vi "CSM_GNSS.vi"(8 "Error In":errorcluster, 11 "Command":string) -> (0 "Error Out":errorcluster, 3 "Response":string)   [LabVIEW 2018]
uses:
  MOKO_LabViewLibrary/MokoLowLevel/MokoLowLovelControl/MLLC_Mode.ctl
  data/CSM_GNSS.ctl
  windows/Environments.ctl
  windows/Equipment.ctl
  windows/Registration.ctl
panel:
  in  "Settings":T5
  in  "Error Code":u32
  in  "Utility Name":string="CSM_GNSS"
  in  "Mode":T6
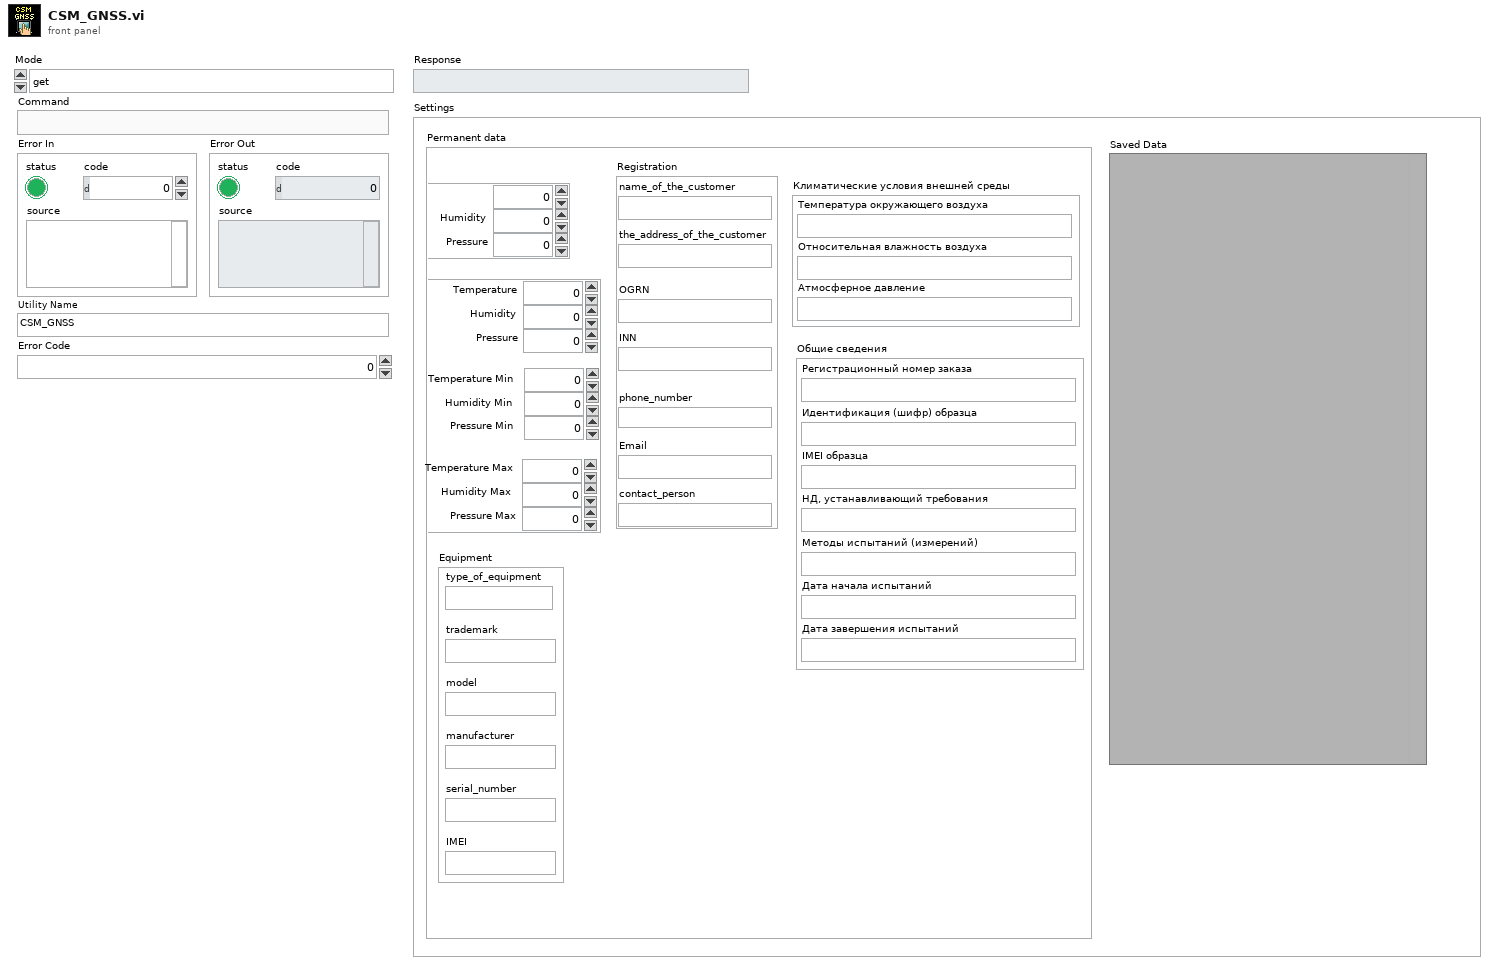
[diagram p1: front panel]
types:
  T1 = typedef "CSM_GNSS.ctl" = cluster{"Environment":cluster{"Temperature":dbl, "Humidity":dbl, "Pressure":dbl}, "Environments":T2, "Equipment":T3, "Registration":T4, "Общие сведения":cluster{"Регистрационный номер заказа":string, "Идентификация (шифр) образца":string, "IMEI образца":string, "НД, устанавливающий требования":string, "Методы испытаний (измерений)":string, "Дата начала испытаний":string, "Дата завершения испытаний":string}, "Климатические условия внешней среды":cluster{"Температура окружающего воздуха":string, "Относительная влажность воздуха":string, "Атмосферное давление":string}}
  T2 = typedef "Environments.ctl" = cluster{"Temperature Min":dbl, "Humidity Min":dbl, "Pressure Min":dbl, "Temperature Max":dbl, "Humidity Max":dbl, "Pressure Max":dbl, "Temperature":dbl, "Humidity":dbl, "Pressure":dbl}
  T3 = typedef "Equipment.ctl" = cluster{"type_of_equipment":string, "trademark":string, "model":string, "manufacturer":string, "serial_number":string, "IMEI":string}
  T4 = typedef "Registration.ctl" = cluster{"name_of_the_customer":string, "the_address_of_the_customer":string, "OGRN":string, "INN":string, "phone_number":string, "Email":string, "contact_person":string}
  T5 = cluster{"Permanent data":T1, "Saved Data":variant}
  T6 = typedef "MLLC_Mode.ctl" = enum16{"get", "set", "close", "Init", "Check"}
  T7 = cluster{"Temperature":dbl, "Humidity":dbl, "Pressure":dbl}
  T8 = typedef "MLLC_Error.ctl" = errorcluster
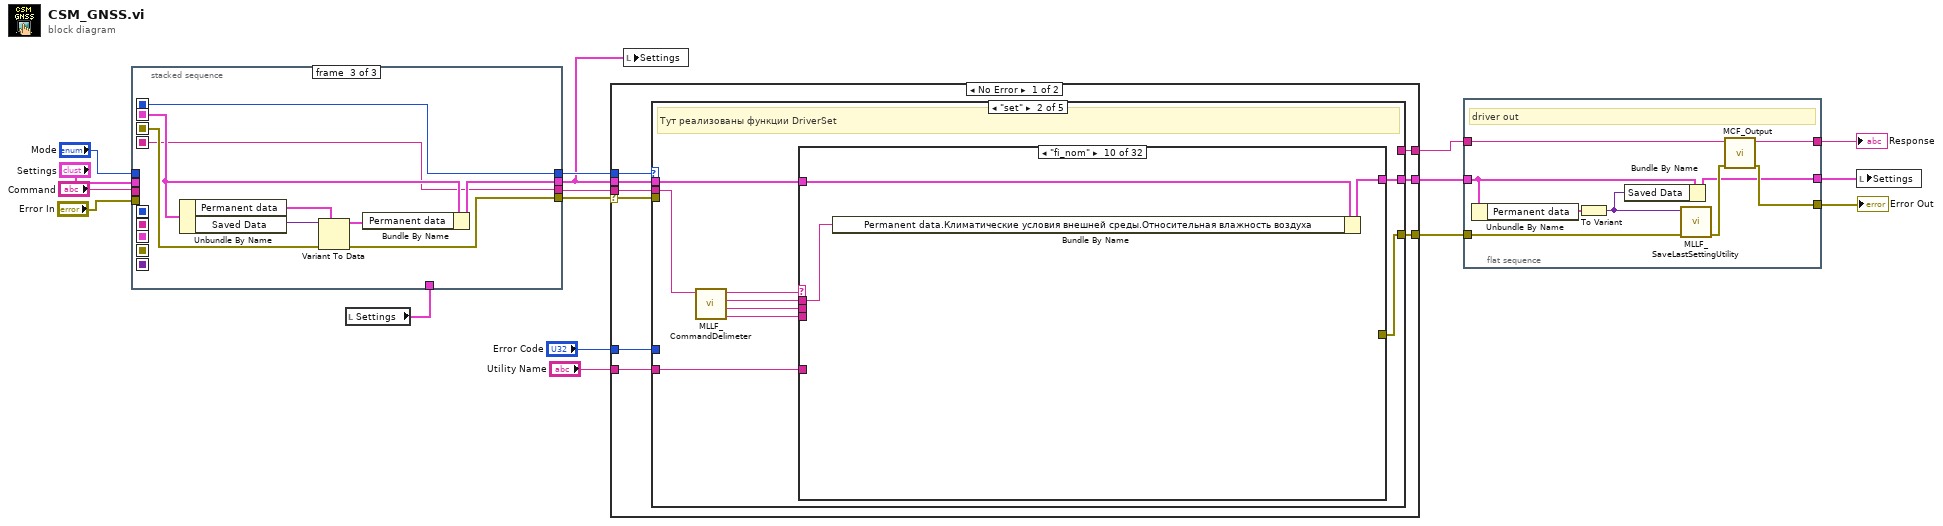
[diagram p0: block diagram]
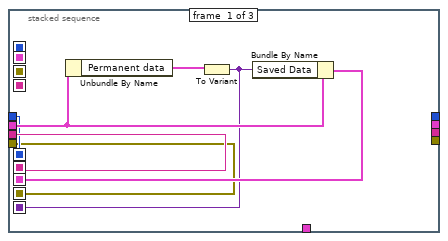
[diagram p2: hidden frame]
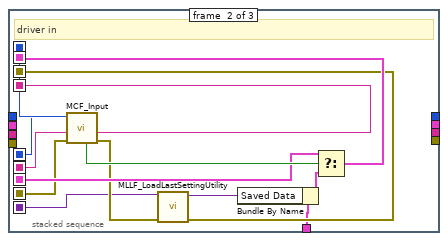
[diagram p3: hidden frame]
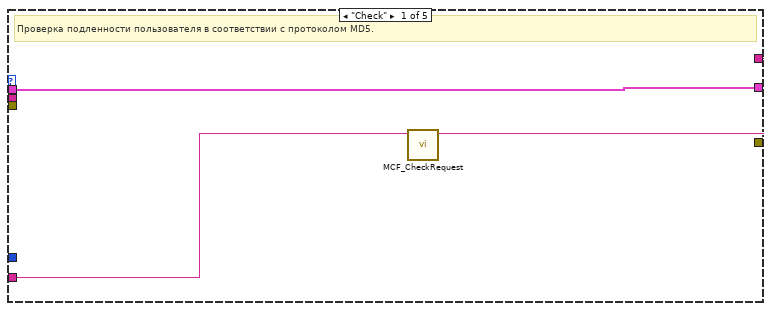
[diagram p4: hidden frame]
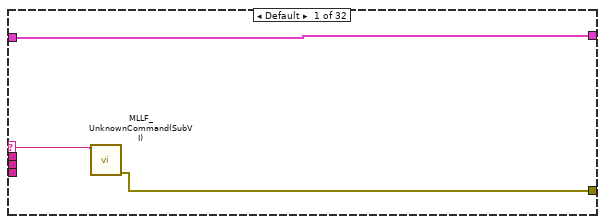
[diagram p5: hidden frame]
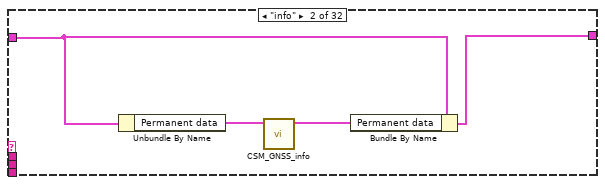
[diagram p6: hidden frame]
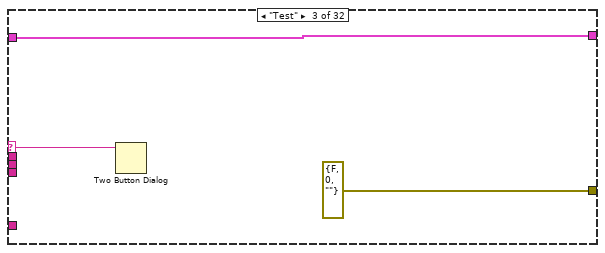
[diagram p7: hidden frame]
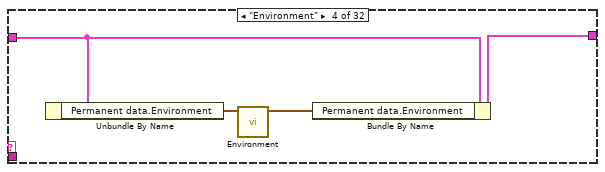
[diagram p8: hidden frame]
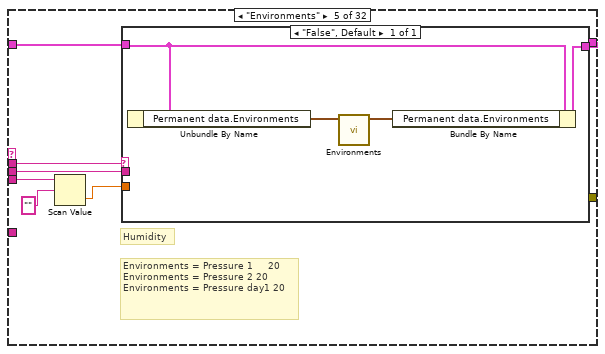
[diagram p9: hidden frame]
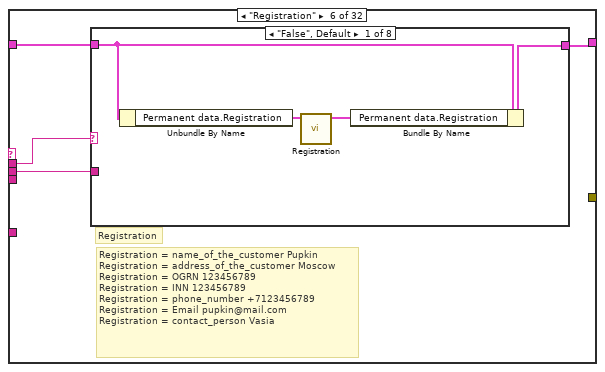
[diagram p10: hidden frame]
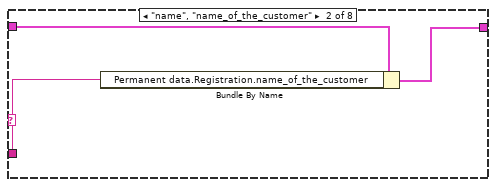
[diagram p11: hidden frame]
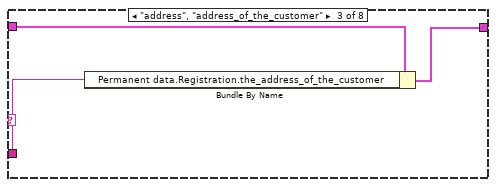
[diagram p12: hidden frame]
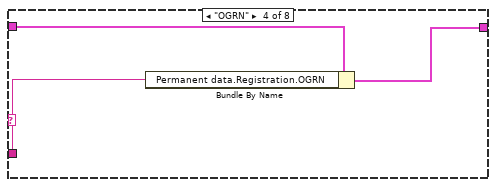
[diagram p13: hidden frame]
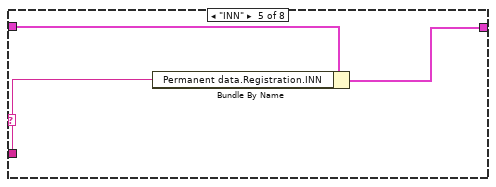
[diagram p14: hidden frame]
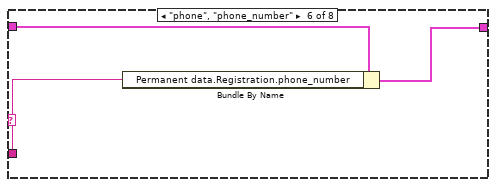
[diagram p15: hidden frame]
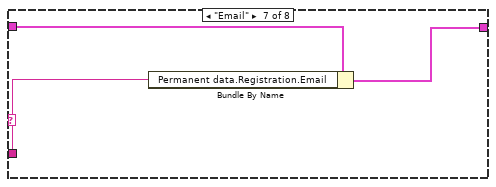
[diagram p16: hidden frame]
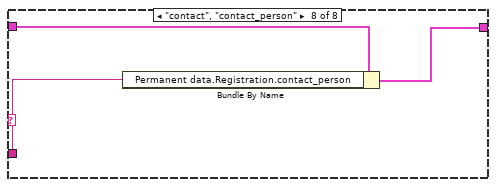
[diagram p17: hidden frame]
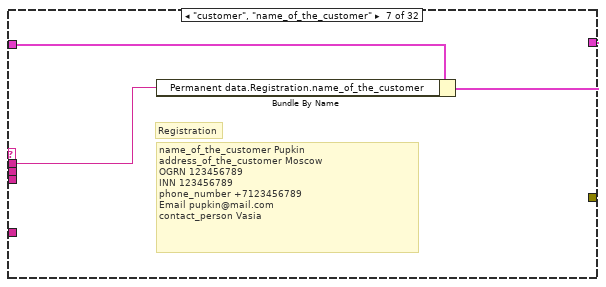
[diagram p18: hidden frame]
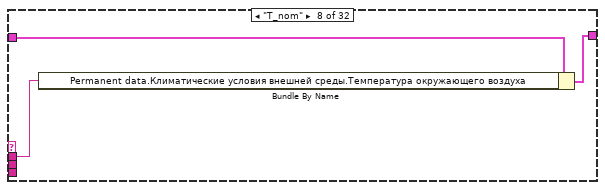
[diagram p19: hidden frame]
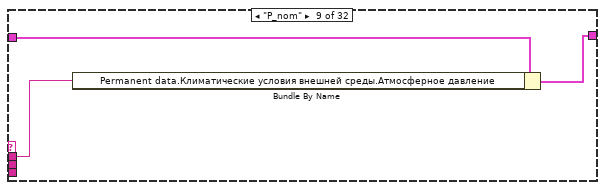
[diagram p20: hidden frame]
diagram:
  n1 = local read "Settings"() -> (w11:T5)
  n2 = stacked-sequence {
    seq-local: [w20 _ _] -> [_ w36 _]
    seq-local: [w19 _ _] -> [_ w37 _]
    seq-local: [w22 _ _] -> [_ w32 _]
    seq-local: [w18 _ _] -> [_ w31 _]
    seq-local: [w21 _ _] -> [_ w26 _]
    seq-local: [_ w27 _] -> [_ _ w43]
    seq-local: [_ w38 _] -> [_ _ w40]
    seq-local: [_ w35 _] -> [_ _ w39]
    seq-local: [_ w34 _] -> [_ _ w44]
    tunnel: "Command" -> [w20 _ _]
    tunnel: "Mode" -> [w19 _ _]
    tunnel: "Error In" -> [w18 _ _]
    tunnel: "Settings" -> [w23 _ _]
    tunnel: w11 -> [_ w25 _]
    tunnel: [_ _ w39] -> w7
    tunnel: [_ _ w42] -> w9
    tunnel: [_ _ w41] -> w8
    tunnel: [_ _ w40] -> w10
    frame #0 {
      n3 = Unbundle By Name(w23) -> ("Permanent data"=w24:T1)
      n4 = To Variant(anything=w24) -> (Variant=w21:variant)
      n5 = Bundle By Name(cluster=w23, "Saved Data"=w21) -> (w22:T5)
    }
    frame #1 {
      # "driver in"
      n6 = call "MCF_Input.vi"("Error In"=w31, "Command in"=w36, "Mode in"=w37) -> ("Error Out"=w30:errorcluster, "Command out"=w35:string, "Mode out"=w38:T6, "Boolean"=w33:bool)  [unwired: 5 in]
      n7 = call "MLLF_LoadLastSettingUtility.vi"("Error In"=w30, "Save data in"=w26) -> ("Error Out"=w27:errorcluster, "Save data out"=w29:variant)  [unwired: 8 in]
      n8 = Bundle By Name(cluster=w25, "Saved Data"=w29) -> (w28:T5)
      n9 = Select(t=w32, s=w33, f=w28) -> (s? t:f=w34:T5)
    }
    frame #2 {
      n10 = Unbundle By Name(w44) -> ("Permanent data"=w45:T1, "Saved Data"=w47:variant)
      n11 = Variant To Data(error in=w43, type=w45, Variant=w47) -> (data=w46:T1, error out=w41:errorcluster)
      n12 = Bundle By Name(cluster=w44, "Permanent data"=w46) -> (w42:T5)
    }
  }
  n13 = case shown="No Error" w8 {
    selector: w8 -> [w52 w346]
    tunnel: [w54 w346] -> w4
    tunnel: w10 -> [w56 _]
    tunnel: [w55 _] -> w6
    tunnel: w7 -> [w53 _]
    tunnel: w9 -> [w49 w345]
    tunnel: "Error Code" -> [w51 _]
    tunnel: "Utility Name" -> [w50 _]
    tunnel: [w48 w345] -> w5
    frame No Error {
      n14 = case shown="\"set\"" w56 {
        tunnel: [w57 _ w221 _ _] -> w55
        tunnel: [_ w67 w223 _ _] -> w54
        tunnel: w53 -> [_ w68 w226 _ _]
        tunnel: w52 -> [_ _ _ _ _]
        tunnel: w51 -> [_ _ _ _ _]
        tunnel: w50 -> [w58 w60 w220 _ _]
        tunnel: w49 -> [w59 w66 w225 _ _]
        tunnel: [w59 w65 w224 _ _] -> w48
        frame "Check" {
          # "Проверка подленности пользователя в соответствии с протоколом MD5."
          n15 = call "MCF_CheckRequest.vi"("Driver Name"=w58) -> ("Output String"=w57:string)  [unwired: 9 in, 1 out]
        }
        frame "set" {
          # "Тут реализованы функции DriverSet"
          n16 = call "MLLF_CommandDelimeter.vi"("command with param"=w68) -> ("param 3"=w61:string, "param 2"=w62:string, "param 1"=w64:string, "command"=w63:string)  [unwired: 6 in, 1 out]
          n17 = case shown="\"fi_nom\"" w63 {
            selector: w63 -> [w70 _ w76 _ _ _ _ _ _ _ _ _ _ _ _ _ _ _ _ _ _ _ _ _ _ _ _ _ _ _ _ _]
            tunnel: [w71 w72 w78 w80 w88 w96 w124 w127 w130 w133 w136 w139 w142 w145 w148 w151 w153 w158 w161 w164 w167 w170 w173 w178 w183 w188 w193 w198 w203 w208 w213 w218] -> w65
            tunnel: w66 -> [w71 w74 w78 w81 w89 w97 w125 w128 w131 w134 w137 w140 w143 w146 w149 w152 w155 w159 w162 w165 w168 w171 w174 w179 w184 w189 w194 w199 w204 w209 w214 w219]
            tunnel: [w69 _ errorcluster {"status"=FALSE, "code"=0, "source"=""} ("error IO") _ _ _ _ _ _ _ _ _ _ _ _ _ _ _ _ _ _ _ _ _ _ _ _ _ _ _ _ _] -> w67
            tunnel: w64 -> [_ _ _ _ w85 w95 w123 w126 w129 w132 w135 w138 w141 w144 w147 w150 _ w157 w160 w163 w166 w169 w172 w175 w180 w185 w190 w195 w200 w205 w210 w215]
            tunnel: w62 -> [_ _ _ _ w84 w94 _ _ _ _ _ _ _ _ _ _ _ _ _ _ _ _ _ _ _ _ _ _ _ _ _ _]
            tunnel: w61 -> [_ _ _ _ w83 _ _ _ _ _ _ _ _ _ _ _ _ _ _ _ _ _ _ _ _ _ _ _ _ _ _ _]
            tunnel: w60 -> [_ _ _ _ _ _ _ _ _ _ _ _ _ _ _ _ _ _ _ _ _ _ _ _ _ _ _ _ _ _ _ _]
            frame Default {
              n18 = call "MLLF_UnknownCommand(SubVI).vi"("Unknown command"=w70) -> ("error out"=w69:errorcluster)  [unwired: 10 in]
            }
            frame "info" {
              n19 = Unbundle By Name(w74) -> ("Permanent data"=w75:T1)
              n20 = call "CSM_GNSS_info.vi"("CSMinfo in"=w75) -> ("CSMinfo out"=w73:T1)  [unwired: 9 in, 1 out]
              n21 = Bundle By Name(cluster=w74, "Permanent data"=w73) -> (w72:T5)
            }
            frame "Test" {
              n22 = Two Button Dialog(message=w76) -> ()  [unwired: 2 in, 1 out]
            }
            frame "Environment" {
              n23 = Unbundle By Name(w81) -> ("Permanent data.Environment"=w82:T7)
              n24 = call "Environment.vi"("Environment in"=w82) -> ("Environment out"=w79:T7)  [unwired: 9 in, 1 out]
              n25 = Bundle By Name(cluster=w81, "Permanent data.Environment"=w79) -> (w80:T5)
            }
            frame "Environments" {
              # "Humidity"
              # "Environments = Pressure 1     20\nEnvironments = Pressure 2 20\nEnvironments = Pressure day1 20"
              n26 = Scan Value(string=w83, format string="") -> (value=w87:dbl)  [unwired: 1 in, 1 out]
              n27 = case shown="\"False\", Default" w85 {
                tunnel: w89 -> [w91]
                tunnel: [w90] -> w88
                tunnel: w87 -> [_]
                tunnel: w84 -> [_]
                frame "False", Default {
                  n28 = Unbundle By Name(w91) -> ("Permanent data.Environments"=w93:T2)
                  n29 = call "Environments.vi"("Environments in"=w93) -> ("Environments out"=w92:T2)  [unwired: 9 in, 1 out]
                  n30 = Bundle By Name(cluster=w91, "Permanent data.Environments"=w92) -> (w90:T5)
                }
              }
            }
            frame "Registration" {
              # "Registration"
              # "Registration = name_of_the_customer Pupkin\nRegistration = address_of_the_customer Moscow\nRegistration = OGRN 123456789\nRegistration = INN 123456789\nRegistration = phone_number +7123456789\nRegistration = Email pupkin@mail.com\nRegistration = contact_person Vasia"
              n31 = case shown="\"False\", Default" w95 {
                tunnel: w97 -> [w100 w104 w107 w110 w113 w116 w119 w122]
                tunnel: [w99 w103 w106 w109 w112 w115 w118 w121] -> w96
                tunnel: w94 -> [_ w102 w105 w108 w111 w114 w117 w120]
                frame "False", Default {
                  n32 = Unbundle By Name(w100) -> ("Permanent data.Registration"=w101:T4)
                  n33 = call "Registration.vi"("Registration in"=w101) -> ("Registration out"=w98:T4)  [unwired: 9 in, 1 out]
                  n34 = Bundle By Name(cluster=w100, "Permanent data.Registration"=w98) -> (w99:T5)
                }
                frame "name", "name_of_the_customer" {
                  n35 = Bundle By Name(cluster=w104, "Permanent data.Registration.name_of_the_customer"=w102) -> (w103:T5)
                }
                frame "address", "address_of_the_customer" {
                  n36 = Bundle By Name(cluster=w107, "Permanent data.Registration.the_address_of_the_customer"=w105) -> (w106:T5)
                }
                frame "OGRN" {
                  n37 = Bundle By Name(cluster=w110, "Permanent data.Registration.OGRN"=w108) -> (w109:T5)
                }
                frame "INN" {
                  n38 = Bundle By Name(cluster=w113, "Permanent data.Registration.INN"=w111) -> (w112:T5)
                }
                frame "phone", "phone_number" {
                  n39 = Bundle By Name(cluster=w116, "Permanent data.Registration.phone_number"=w114) -> (w115:T5)
                }
                frame "Email" {
                  n40 = Bundle By Name(cluster=w119, "Permanent data.Registration.Email"=w117) -> (w118:T5)
                }
                frame "contact", "contact_person" {
                  n41 = Bundle By Name(cluster=w122, "Permanent data.Registration.contact_person"=w120) -> (w121:T5)
                }
              }
            }
            frame "customer", "name_of_the_customer" {
              # "Registration"
              # "name_of_the_customer Pupkin\naddress_of_the_customer Moscow\nOGRN 123456789\nINN 123456789\nphone_number +7123456789\nEmail pupkin@mail.com\ncontact_person Vasia"
              n42 = Bundle By Name(cluster=w125, "Permanent data.Registration.name_of_the_customer"=w123) -> (w124:T5)
            }
            frame "T_nom" {
              n43 = Bundle By Name(cluster=w128, "Permanent data.Климатические условия внешней среды.Температура окружающего воздуха"=w126) -> (w127:T5)
            }
            frame "P_nom" {
              n44 = Bundle By Name(cluster=w131, "Permanent data.Климатические условия внешней среды.Атмосферное давление"=w129) -> (w130:T5)
            }
            frame "fi_nom" {
              n45 = Bundle By Name(cluster=w134, "Permanent data.Климатические условия внешней среды.Относительная влажность воздуха"=w132) -> (w133:T5)
            }
            frame "address", "the_address_of_the_customer" {
              # "Registration"
              # "name_of_the_customer Pupkin\naddress_of_the_customer Moscow\nOGRN 123456789\nINN 123456789\nphone_number +7123456789\nEmail pupkin@mail.com\ncontact_person Vasia"
              n46 = Bundle By Name(cluster=w137, "Permanent data.Registration.the_address_of_the_customer"=w135) -> (w136:T5)
            }
            frame "OGRN" {
              # "Registration"
              # "name_of_the_customer Pupkin\naddress_of_the_customer Moscow\nOGRN 123456789\nINN 123456789\nphone_number +7123456789\nEmail pupkin@mail.com\ncontact_person Vasia"
              n47 = Bundle By Name(cluster=w140, "Permanent data.Registration.OGRN"=w138) -> (w139:T5)
            }
            frame "INN" {
              # "Registration"
              # "name_of_the_customer Pupkin\naddress_of_the_customer Moscow\nOGRN 123456789\nINN 123456789\nphone_number +7123456789\nEmail pupkin@mail.com\ncontact_person Vasia"
              n48 = Bundle By Name(cluster=w143, "Permanent data.Registration.INN"=w141) -> (w142:T5)
            }
            frame "phone", "phone_number" {
              # "Registration"
              # "name_of_the_customer Pupkin\naddress_of_the_customer Moscow\nOGRN 123456789\nINN 123456789\nphone_number +7123456789\nEmail pupkin@mail.com\ncontact_person Vasia"
              n49 = Bundle By Name(cluster=w146, "Permanent data.Registration.phone_number"=w144) -> (w145:T5)
            }
            frame "Email" {
              # "Registration"
              # "name_of_the_customer Pupkin\naddress_of_the_customer Moscow\nOGRN 123456789\nINN 123456789\nphone_number +7123456789\nEmail pupkin@mail.com\ncontact_person Vasia"
              n50 = Bundle By Name(cluster=w149, "Permanent data.Registration.Email"=w147) -> (w148:T5)
            }
            frame "contact", "contact_person" {
              # "Registration"
              # "name_of_the_customer Pupkin\naddress_of_the_customer Moscow\nOGRN 123456789\nINN 123456789\nphone_number +7123456789\nEmail pupkin@mail.com\ncontact_person Vasia"
              n51 = Bundle By Name(cluster=w152, "Permanent data.Registration.contact_person"=w150) -> (w151:T5)
            }
            frame "Equipment" {
              n52 = Unbundle By Name(w155) -> ("Permanent data.Equipment"=w156:T3)
              n53 = call "Equipment.vi"("Equipment in"=w156) -> ("Equipment out"=w154:T3)  [unwired: 9 in, 1 out]
              n54 = Bundle By Name(cluster=w155, "Permanent data.Equipment"=w154) -> (w153:T5)
            }
            frame "type_of_equipment" {
              # "Equipment"
              # "type_of_equipment Reciever\ntrademark Roga&Kopyta\nmodel Model_1\nmanufacturer Roga&Kopyta\nserial_number 123456789\nIMEI 55613216568486483465"
              n55 = Bundle By Name(cluster=w159, "Permanent data.Equipment.type_of_equipment"=w157) -> (w158:T5)
            }
            frame "trademark" {
              # "Equipment"
              # "type_of_equipment Reciever\ntrademark Roga&Kopyta\nmodel Model_1\nmanufacturer Roga&Kopyta\nserial_number 123456789\nIMEI 55613216568486483465"
              n56 = Bundle By Name(cluster=w162, "Permanent data.Equipment.trademark"=w160) -> (w161:T5)
            }
            frame "model" {
              # "Equipment"
              # "type_of_equipment Reciever\ntrademark Roga&Kopyta\nmodel Model_1\nmanufacturer Roga&Kopyta\nserial_number 123456789\nIMEI 55613216568486483465"
              n57 = Bundle By Name(cluster=w165, "Permanent data.Equipment.model"=w163) -> (w164:T5)
            }
            frame "manufacturer" {
              # "Equipment"
              # "type_of_equipment Reciever\ntrademark Roga&Kopyta\nmodel Model_1\nmanufacturer Roga&Kopyta\nserial_number 123456789\nIMEI 55613216568486483465"
              n58 = Bundle By Name(cluster=w168, "Permanent data.Equipment.manufacturer"=w166) -> (w167:T5)
            }
            frame "serial_number" {
              # "Equipment"
              # "type_of_equipment Reciever\ntrademark Roga&Kopyta\nmodel Model_1\nmanufacturer Roga&Kopyta\nserial_number 123456789\nIMEI 55613216568486483465"
              n59 = Bundle By Name(cluster=w171, "Permanent data.Equipment.serial_number"=w169) -> (w170:T5)
            }
            frame "IMEI" {
              # "Equipment"
              # "type_of_equipment Reciever\ntrademark Roga&Kopyta\nmodel Model_1\nmanufacturer Roga&Kopyta\nserial_number 123456789\nIMEI 55613216568486483465"
              n60 = Bundle By Name(cluster=w174, "Permanent data.Equipment.IMEI"=w172) -> (w173:T5)
            }
            frame "Temperature" {
              # "Enviroments"
              # "Temperature 25\nHumidity 50\nPressure 100\nTemperature_min 25\nHumidity_min 50\nPressure_min 100\nTemperature_max 25\nHumidity_max 50\nPressure_max 100"
              n61 = Scan Value(string=w175, format string="") -> (value=w177:dbl)  [unwired: 1 in, 1 out]
              n62 = Bundle By Name(cluster=w179, "Permanent data.Environment.Temperature"=w177) -> (w178:T5)
            }
            frame "Humidity" {
              # "Enviroments"
              # "Temperature 25\nHumidity 50\nPressure 100\nTemperature_min 25\nHumidity_min 50\nPressure_min 100\nTemperature_max 25\nHumidity_max 50\nPressure_max 100"
              n63 = Scan Value(string=w180, format string="") -> (value=w182:dbl)  [unwired: 1 in, 1 out]
              n64 = Bundle By Name(cluster=w184, "Permanent data.Environment.Humidity"=w182) -> (w183:T5)
            }
            frame "Pressure" {
              # "Enviroments"
              # "Temperature 25\nHumidity 50\nPressure 100\nTemperature_min 25\nHumidity_min 50\nPressure_min 100\nTemperature_max 25\nHumidity_max 50\nPressure_max 100"
              n65 = Scan Value(string=w185, format string="") -> (value=w187:dbl)  [unwired: 1 in, 1 out]
              n66 = Bundle By Name(cluster=w189, "Permanent data.Environment.Pressure"=w187) -> (w188:T5)
            }
            frame "Temperature_min", "TemperatureMin" {
              # "Enviroments"
              # "Temperature 25\nHumidity 50\nPressure 100\nTemperature_min 25\nHumidity_min 50\nPressure_min 100\nTemperature_max 25\nHumidity_max 50\nPressure_max 100"
              n67 = Scan Value(string=w190, format string="") -> (value=w192:dbl)  [unwired: 1 in, 1 out]
              n68 = Bundle By Name(cluster=w194, "Permanent data.Environments.Temperature Min"=w192) -> (w193:T5)
            }
            frame "Humidity_min", "HumidityMin" {
              # "Enviroments"
              # "Temperature 25\nHumidity 50\nPressure 100\nTemperature_min 25\nHumidity_min 50\nPressure_min 100\nTemperature_max 25\nHumidity_max 50\nPressure_max 100"
              n69 = Scan Value(string=w195, format string="") -> (value=w197:dbl)  [unwired: 1 in, 1 out]
              n70 = Bundle By Name(cluster=w199, "Permanent data.Environments.Humidity Min"=w197) -> (w198:T5)
            }
            frame "Pressure_min", "PressureMin" {
              # "Enviroments"
              # "Temperature 25\nHumidity 50\nPressure 100\nTemperature_min 25\nHumidity_min 50\nPressure_min 100\nTemperature_max 25\nHumidity_max 50\nPressure_max 100"
              n71 = Scan Value(string=w200, format string="") -> (value=w202:dbl)  [unwired: 1 in, 1 out]
              n72 = Bundle By Name(cluster=w204, "Permanent data.Environments.Pressure Min"=w202) -> (w203:T5)
            }
            frame "Temperature_max", "TemperatureMax" {
              # "Enviroments"
              # "Temperature 25\nHumidity 50\nPressure 100\nTemperature_min 25\nHumidity_min 50\nPressure_min 100\nTemperature_max 25\nHumidity_max 50\nPressure_max 100"
              n73 = Scan Value(string=w205, format string="") -> (value=w207:dbl)  [unwired: 1 in, 1 out]
              n74 = Bundle By Name(cluster=w209, "Permanent data.Environments.Temperature Max"=w207) -> (w208:T5)
            }
            frame "Humidity_max", "HumidityMax" {
              # "Enviroments"
              # "Temperature 25\nHumidity 50\nPressure 100\nTemperature_min 25\nHumidity_min 50\nPressure_min 100\nTemperature_max 25\nHumidity_max 50\nPressure_max 100"
              n75 = Scan Value(string=w210, format string="") -> (value=w212:dbl)  [unwired: 1 in, 1 out]
              n76 = Bundle By Name(cluster=w214, "Permanent data.Environments.Humidity Max"=w212) -> (w213:T5)
            }
            frame "Pressure_max", "PressureMax" {
              # "Enviroments"
              # "Temperature 25\nHumidity 50\nPressure 100\nTemperature_min 25\nHumidity_min 50\nPressure_min 100\nTemperature_max 25\nHumidity_max 50\nPressure_max 100"
              n77 = Scan Value(string=w215, format string="") -> (value=w217:dbl)  [unwired: 1 in, 1 out]
              n78 = Bundle By Name(cluster=w219, "Permanent data.Environments.Pressure Max"=w217) -> (w218:T5)
            }
          }
        }
        frame "get" {
          # "Тут реализованы функции DriverGet"
          n79 = call "MLLF_CommandDelimeter.vi"("command with param"=w226) -> ("command"=w222:string)  [unwired: 6 in, 4 out]
          n80 = case shown="\"P_nom\"" w222 {
            selector: w222 -> [w228 _ _ _ _ _ _ _ _ _ _ _ _ _ _ _ _ _ _ _ _ _ _ _ _ _ _ _ _ _ _ _]
            tunnel: w225 -> [w229 w235 w240 w243 w249 w255 w261 w267 w273 w279 w285 w292 w294 w296 w298 w300 w302 w304 w306 w308 w311 w314 w317 w320 w323 w326 w329 w332 w335 w338 w341 w344]
            tunnel: [w229 w235 w240 w243 w249 w255 w261 w267 w273 w279 w285 w292 w294 w296 w298 w300 w302 w304 w306 w308 w311 w314 w317 w320 w323 w326 w329 w332 w335 w338 w341 w344] -> w224
            tunnel: [_ w230 w236 w242 w248 w254 w260 w266 w272 w278 w284 w290 w293 w295 w297 w299 w301 w303 w305 w307 w310 w313 w316 w319 w322 w325 w328 w331 w334 w337 w340 w343] -> w221
            tunnel: [w227 _ _ _ _ _ _ _ _ _ _ _ _ _ _ _ _ _ _ _ _ _ _ _ _ _ _ _ _ _ _ _] -> w223
            tunnel: w220 -> [_ _ _ _ _ _ _ _ _ _ _ _ _ _ _ _ _ _ _ _ _ _ _ _ _ _ _ _ _ _ _ _]
            frame Default {
              n81 = call "MLLF_UnknownCommand(SubVI).vi"("Unknown command"=w228) -> ("error out"=w227:errorcluster)  [unwired: 10 in]
            }
            frame "Test" {
              n82 = Two Button Dialog(message="Test") -> (T button?=w234:bool)  [unwired: 2 in]
              n83 = Select(t="True" ("string"), s=w234, f="False" ("string")) -> (s? t:f=w230:string)
            }
            frame "Temperature" {
              n84 = Unbundle By Name(w240) -> ("Permanent data.Environment.Temperature"=w241:dbl)
              n85 = Format Value(value (0)=w241) -> (output string=w239:string)  [unwired: 2 in]
              n86 = Search and Replace String(input string=w239, search string=",", replace string="." ("replace string (\"\")")) -> (result string=w236:string)  [unwired: 5 in, 3 out]
            }
            frame "Humidity" {
              n87 = Unbundle By Name(w243) -> ("Permanent data.Environment.Humidity"=w247:dbl)
              n88 = Format Value(value (0)=w247) -> (output string=w246:string)  [unwired: 2 in]
              n89 = Search and Replace String(input string=w246, search string=",", replace string="." ("replace string (\"\")")) -> (result string=w242:string)  [unwired: 5 in, 3 out]
            }
            frame "Pressure" {
              n90 = Unbundle By Name(w249) -> ("Permanent data.Environment.Pressure"=w253:dbl)
              n91 = Format Value(value (0)=w253) -> (output string=w252:string)  [unwired: 2 in]
              n92 = Search and Replace String(input string=w252, search string=",", replace string="." ("replace string (\"\")")) -> (result string=w248:string)  [unwired: 5 in, 3 out]
            }
            frame "Temperature_min", "TemperatureMin" {
              n93 = Unbundle By Name(w255) -> ("Permanent data.Environments.Temperature Min"=w259:dbl)
              n94 = Format Value(value (0)=w259) -> (output string=w258:string)  [unwired: 2 in]
              n95 = Search and Replace String(input string=w258, search string=",", replace string="." ("replace string (\"\")")) -> (result string=w254:string)  [unwired: 5 in, 3 out]
            }
            frame "Humidity_min", "HumidityMin" {
              n96 = Unbundle By Name(w261) -> ("Permanent data.Environments.Humidity Min"=w265:dbl)
              n97 = Format Value(value (0)=w265) -> (output string=w264:string)  [unwired: 2 in]
              n98 = Search and Replace String(input string=w264, search string=",", replace string="." ("replace string (\"\")")) -> (result string=w260:string)  [unwired: 5 in, 3 out]
            }
            frame "Pressure_min", "PressureMin" {
              n99 = Unbundle By Name(w267) -> ("Permanent data.Environments.Pressure Min"=w271:dbl)
              n100 = Format Value(value (0)=w271) -> (output string=w270:string)  [unwired: 2 in]
              n101 = Search and Replace String(input string=w270, search string=",", replace string="." ("replace string (\"\")")) -> (result string=w266:string)  [unwired: 5 in, 3 out]
            }
            frame "Temperature_max", "TemperatureMax" {
              n102 = Unbundle By Name(w273) -> ("Permanent data.Environments.Temperature Max"=w277:dbl)
              n103 = Format Value(value (0)=w277) -> (output string=w276:string)  [unwired: 2 in]
              n104 = Search and Replace String(input string=w276, search string=",", replace string="." ("replace string (\"\")")) -> (result string=w272:string)  [unwired: 5 in, 3 out]
            }
            frame "Humidity_max", "HumidityMax" {
              n105 = Unbundle By Name(w279) -> ("Permanent data.Environments.Humidity Max"=w283:dbl)
              n106 = Format Value(value (0)=w283) -> (output string=w282:string)  [unwired: 2 in]
              n107 = Search and Replace String(input string=w282, search string=",", replace string="." ("replace string (\"\")")) -> (result string=w278:string)  [unwired: 5 in, 3 out]
            }
            frame "Pressure_max", "PressureMax" {
              n108 = Unbundle By Name(w285) -> ("Permanent data.Environments.Pressure Max"=w289:dbl)
              n109 = Format Value(value (0)=w289) -> (output string=w288:string)  [unwired: 2 in]
              n110 = Search and Replace String(input string=w288, search string=",", replace string="." ("replace string (\"\")")) -> (result string=w284:string)  [unwired: 5 in, 3 out]
            }
            frame "customer", "name_of_the_customer" {
              n111 = Unbundle By Name(w292) -> ("Permanent data.Registration.name_of_the_customer"=w291:string)
              n112 = call "MLLF_ReplaceTwoQuotesWithOne.vi"("String in 2"=w291) -> ("Result string"=w290:string)  [unwired: 7 in, 3 out]
            }
            frame "RegistrationID" {
              n113 = Unbundle By Name(w294) -> ("Permanent data.Общие сведения.Регистрационный номер заказа"=w293:string)
            }
            frame "cipher" {
              n114 = Unbundle By Name(w296) -> ("Permanent data.Общие сведения.Идентификация (шифр) образца"=w295:string)
            }
            frame "IMEI" {
              n115 = Unbundle By Name(w298) -> ("Permanent data.Общие сведения.IMEI образца"=w297:string)
            }
            frame "start_test_date" {
              n116 = Unbundle By Name(w300) -> ("Permanent data.Общие сведения.Дата начала испытаний"=w299:string)
            }
            frame "completion_test_date" {
              n117 = Unbundle By Name(w302) -> ("Permanent data.Общие сведения.Дата завершения испытаний"=w301:string)
            }
            frame "T_nom" {
              n118 = Unbundle By Name(w304) -> ("Permanent data.Климатические условия внешней среды.Температура окружающего воздуха"=w303:string)
            }
            frame "fi_nom" {
              n119 = Unbundle By Name(w306) -> ("Permanent data.Климатические условия внешней среды.Относительная влажность воздуха"=w305:string)
            }
            frame "P_nom" {
              n120 = Unbundle By Name(w308) -> ("Permanent data.Климатические условия внешней среды.Атмосферное давление"=w307:string)
            }
            frame "address", "the_address_of_the_customer" {
              n121 = Unbundle By Name(w311) -> ("Permanent data.Registration.the_address_of_the_customer"=w309:string)
              n122 = call "MLLF_ReplaceTwoQuotesWithOne.vi"("String in"=w309) -> ("Result string"=w310:string)  [unwired: 7 in, 3 out]
            }
            frame "OGRN" {
              n123 = Unbundle By Name(w314) -> ("Permanent data.Registration.OGRN"=w312:string)
              n124 = call "MLLF_ReplaceTwoQuotesWithOne.vi"("String in"=w312) -> ("Result string"=w313:string)  [unwired: 7 in, 3 out]
            }
            frame "INN" {
              n125 = Unbundle By Name(w317) -> ("Permanent data.Registration.INN"=w315:string)
              n126 = call "MLLF_ReplaceTwoQuotesWithOne.vi"("String in"=w315) -> ("Result string"=w316:string)  [unwired: 7 in, 3 out]
            }
            frame "phone", "phone_number" {
              n127 = Unbundle By Name(w320) -> ("Permanent data.Registration.phone_number"=w318:string)
              n128 = call "MLLF_ReplaceTwoQuotesWithOne.vi"("String in"=w318) -> ("Result string"=w319:string)  [unwired: 7 in, 3 out]
            }
            frame "Email" {
              n129 = Unbundle By Name(w323) -> ("Permanent data.Registration.Email"=w321:string)
              n130 = call "MLLF_ReplaceTwoQuotesWithOne.vi"("String in"=w321) -> ("Result string"=w322:string)  [unwired: 7 in, 3 out]
            }
            frame "contact", "contact_person" {
              n131 = Unbundle By Name(w326) -> ("Permanent data.Registration.contact_person"=w324:string)
              n132 = call "MLLF_ReplaceTwoQuotesWithOne.vi"("String in"=w324) -> ("Result string"=w325:string)  [unwired: 7 in, 3 out]
            }
            frame "type_of_equipment" {
              n133 = Unbundle By Name(w329) -> ("Permanent data.Equipment.type_of_equipment"=w327:string)
              n134 = call "MLLF_ReplaceTwoQuotesWithOne.vi"("String in"=w327) -> ("Result string"=w328:string)  [unwired: 7 in, 3 out]
            }
            frame "trademark" {
              n135 = Unbundle By Name(w332) -> ("Permanent data.Equipment.trademark"=w330:string)
              n136 = call "MLLF_ReplaceTwoQuotesWithOne.vi"("String in"=w330) -> ("Result string"=w331:string)  [unwired: 7 in, 3 out]
            }
            frame "model" {
              n137 = Unbundle By Name(w335) -> ("Permanent data.Equipment.model"=w333:string)
              n138 = call "MLLF_ReplaceTwoQuotesWithOne.vi"("String in"=w333) -> ("Result string"=w334:string)  [unwired: 7 in, 3 out]
            }
            frame "manufacturer" {
              n139 = Unbundle By Name(w338) -> ("Permanent data.Equipment.manufacturer"=w336:string)
              n140 = call "MLLF_ReplaceTwoQuotesWithOne.vi"("String in"=w336) -> ("Result string"=w337:string)  [unwired: 7 in, 3 out]
            }
            frame "serial_number" {
              n141 = Unbundle By Name(w341) -> ("Permanent data.Equipment.serial_number"=w339:string)
              n142 = call "MLLF_ReplaceTwoQuotesWithOne.vi"("String in"=w339) -> ("Result string"=w340:string)  [unwired: 7 in, 3 out]
            }
            frame "IMEI_1" {
              n143 = Unbundle By Name(w344) -> ("Permanent data.Equipment.IMEI"=w342:string)
              n144 = call "MLLF_ReplaceTwoQuotesWithOne.vi"("String in"=w342) -> ("Result string"=w343:string)  [unwired: 7 in, 3 out]
            }
          }
        }
        frame "close" {
        }
        frame "Init" {
        }
      }
    }
    frame Error {
    }
  }
  n145 = local write "Settings"(w9) -> ()
  n146 = flat-sequence {
    tunnel: [w355] -> w1
    tunnel: [w354] -> w3
    tunnel: w6 -> [w353]
    tunnel: w4 -> [w352]
    tunnel: w5 -> [w348]
    tunnel: [w350] -> w2
    frame #0 {
      # "driver out"
      n147 = Unbundle By Name(w348) -> ("Permanent data"=w347:T1)
      n148 = To Variant(anything=w347) -> (Variant=w349:variant)
      n149 = Bundle By Name(cluster=w348, "Saved Data"=w349) -> (w350:T5)
      n150 = call "MLLF_SaveLastSettingUtility.vi"("error in"=w352, "Saved Data"=w349) -> ("error out"=w351:T8)  [unwired: 8 in, 1 out]
      n151 = call "MCF_Output.vi"("Error In"=w351, "Input"=w353) -> ("Error Out"=w354:errorcluster, "Output"=w355:string)  [unwired: 8 in]
    }
  }
  n152 = local write "Settings"(w2) -> ()
  "Response" <- w1
  "Error Out" <- w3
